vi "Untitled 2.vi"() -> ()   [LabVIEW 2020]
uses:
  Classes/Controller/Controller.lvclass
panel:
  out "Calibrated Results (bond pad pcb)":sgl[][](array[numeric]) format="%.2f"
  in  "Stop (F)":bool
  out "Image Out":T1(plugin-control)
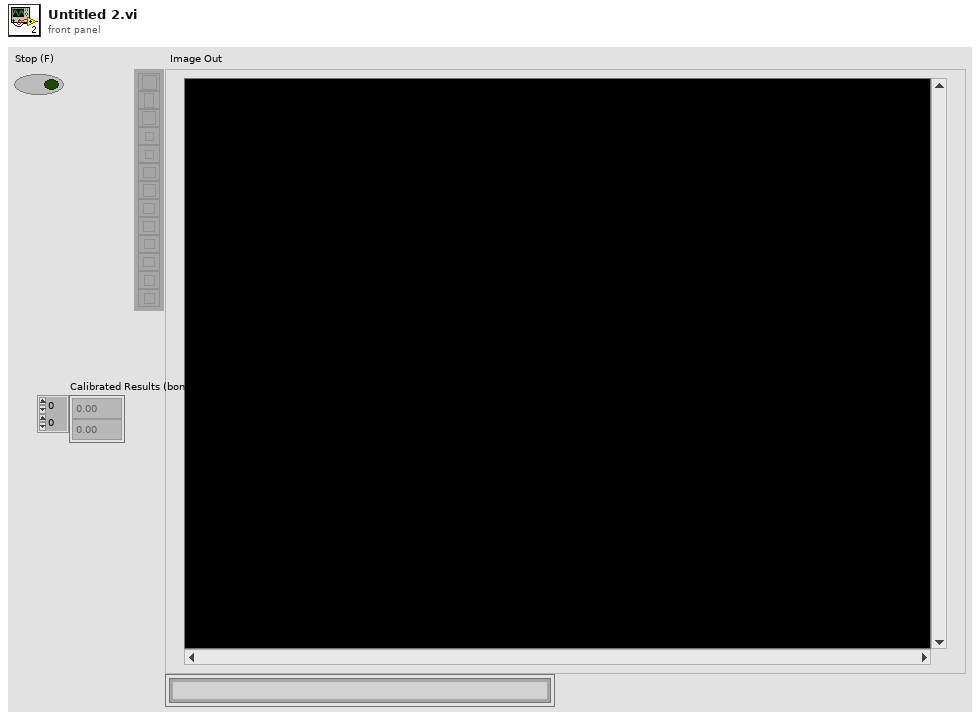
[diagram p1: front panel]
types:
  T1 = typedef "IMAQ Image.ctl" = refnum<image>
  T2 = typedef "Controller.lvclass/Controllers.ctl" = cluster{"I-O.lvclass":refnum<class "I-O.lvclass">, "Dispenser.lvclass":refnum<class "Dispenser.lvclass">, "Gantry":refnum<k24>}
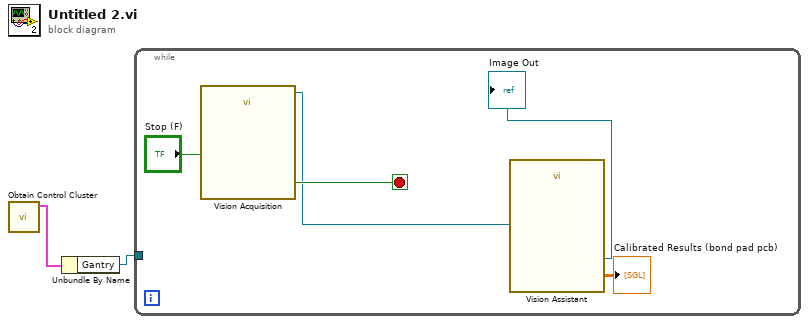
[diagram p0: block diagram]
diagram:
  n1 = call "Obtain Control Cluster.vi"() -> ("Control Out"=w2:T2)  [unwired: 11 in]
  n2 = Unbundle By Name(w2) -> ("Gantry"=w1:refnum<k24>)
  n3 = while {
    tunnel: w1 -> [_]
    stop <- w6 stop-if-true
    n4 = call "Vision Acquisition"("Stop (F)"="Stop (F)") -> ("Image Out"=w5:T1, "Stopped"=w6:bool)  [unwired: 24 in, 1 out]
    n5 = call "Vision Assistant"("Image In"=w5) -> ("Image Out"=→"Image Out":T1, "Calibrated Results (bond pad pcb)"=→"Calibrated Results (bond pad pcb)":sgl[][])  [unwired: 24 in, 1 out]
  }
